vi "oa_Convert Vector Signal View.vi"(6 "view":T1={"dB on? (T)"=FALSE, "unwrap phase? (T)"=TRUE, "unit in degree? (T)"=TRUE}, 10 "phase":dbl[](array[numeric]) format="%.2f", 11 "magnitude":dbl[](array[numeric]) format="%.2f") -> (2 "phase out":dbl[](array[numeric]) format="%.2f", 3 "magnitude out":dbl[](array[numeric]) format="%.2f")   [LabVIEW 2017]
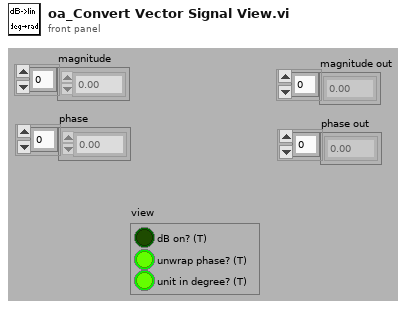
[diagram p1: front panel]
types:
  T1 = cluster{"dB on? (T)":bool, "unwrap phase? (T)":bool, "unit in degree? (T)":bool}
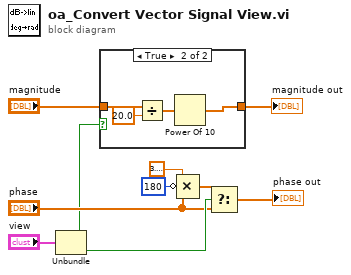
[diagram p0: block diagram]
diagram:
  n1 = Unbundle("view") -> ("dB on? (T)"=w3:bool, "unit in degree? (T)"=w7:bool)  [unwired: 1 out]
  n2 = case shown="True" w3 {
    tunnel: "magnitude" -> [w11 w15]
    tunnel: [w11 w12] -> w1
    frame False {
    }
    frame True {
      n3 = Divide(x=w15, y=20.0) -> (x/y=w13:dbl[])
      n4 = Power Of 10(x=w13) -> (10^x=w12:dbl[])
    }
  }
  "magnitude out" <- w1
  n5 = Compound Arithmetic op=MULTIPLY(3.141592653589793, invert 180, "phase") -> (w10:dbl[])
  n6 = Select(t=w10, s=w7, f="phase") -> (s? t:f=→"phase out":dbl[])
